vi "Setup default numerics.vi"(7 "References":refnum<vi>[](array[refnum]), 8 "error in (no error)":errorcluster, 9 "Property Values":dbl[](array[numeric]), 10 "Property Names":string[](array[string]), 11 "Item Ref In":T1 format="%.0x") -> (0 "error out":errorcluster, 3 "Item Ref out":T1 format="%.0x")   [LabVIEW 2023, in "Embedded TDMS Logger System Explorer.lvlib"]
uses:
  <vilib>/NI VeriStand/Custom Device API/Custom Device Item Ref.ctl
  Embedded TDMS Logger System Explorer.lvlib
  <vilib>/NI VeriStand/Custom Device API/Custom Device API.lvlib
  <vilib>/NI VeriStand/Custom Device API/Get Item Property (Double).vi
  <vilib>/NI VeriStand/Custom Device API/Set Item Property (Double).vi
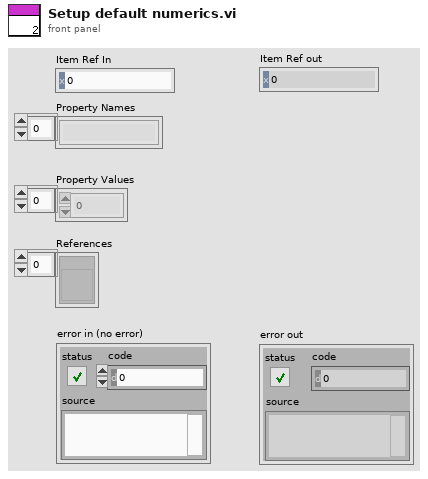
[diagram p1: front panel]
types:
  T1 = typedef "Custom Device API.lvlib/Custom Device Item Ref.ctl" = u64
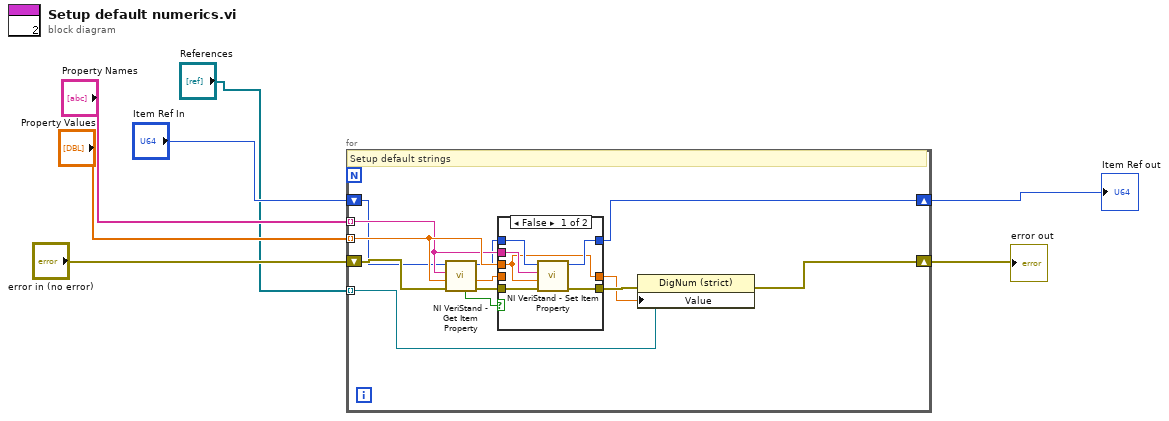
[diagram p0: block diagram]
diagram:
  n1 = for {
    tunnel: "Property Names" -> [w14] mode=indexing
    tunnel: "Property Values" -> [w16] mode=indexing
    shift-right: [w17] -> w3
    shift-left: "error in (no error)" -> [w12]
    shift-right: [w20] -> w6
    shift-left: "Item Ref In" -> [w11]
    tunnel: "References" -> [w19] mode=indexing
    # "Setup default strings"
    n2 = call-poly <vilib>:"NI VeriStand - Get Item Property.vi"("error in (no error)"=w12, "Default Value"=w16, "Property Name"=w14, "Item Ref in"=w11) -> ("error out"=w13:errorcluster, "Value"=w9:dbl, "Item Ref out"=w10:T1, "Found?"=w15:bool)  [unwired: 4 in]
    n3 = case shown="False" w15 {
      tunnel: [w26 w29] -> w20
      tunnel: w10 -> [w25 w29]
      tunnel: [w24 w28] -> w18
      tunnel: w16 -> [w21 _]
      tunnel: w14 -> [w23 _]
      tunnel: w13 -> [w22 w28]
      tunnel: w9 -> [_ w27]
      tunnel: [w21 w27] -> w8
      frame False {
        n4 = call-poly <vilib>:"NI VeriStand - Set Item Property.vi"("error in (no error)"=w22, "Value"=w21, "Property Name"=w23, "Item Ref in"=w25) -> ("error out"=w24:errorcluster, "Item Ref out"=w26:T1)  [unwired: 5 in, 1 out]
      }
      frame True {
      }
    }
    n5 = property class="DigNum (strict)"(reference=w19, error in=w18, "Value"=w8) -> (error out=w17:errorcluster)  [unwired: 1 out]
  }
  "Item Ref out" <- w6
  "error out" <- w3
